vi "sub_check_and_autocreate_channel.vi"(8 "error in (no error)":errorcluster, 9 "daq.io Device Channel Label":string, 10 "daq.io Device Channel Key to write to":string, 11 "daq.io type in in":T1) -> (0 "error out":errorcluster, 1 "channel ID":string, 3 "daq.io type out":T1)   [LabVIEW 2013, in "daqio minimal.lvlib"]
doc: "This VI autocreates a new channel type if required."
uses:
  daqio minimal.lvlib
  _typedefs/daqio-Type.ctl
  <vilib>/httpClient/ClientHandle.ctl
  _typedefs/FGV_commands.ctl
  _typedefs/daqio-Channel-Type.ctl
  <vilib>/httpClient/LabVIEWHTTPClient.lvlib
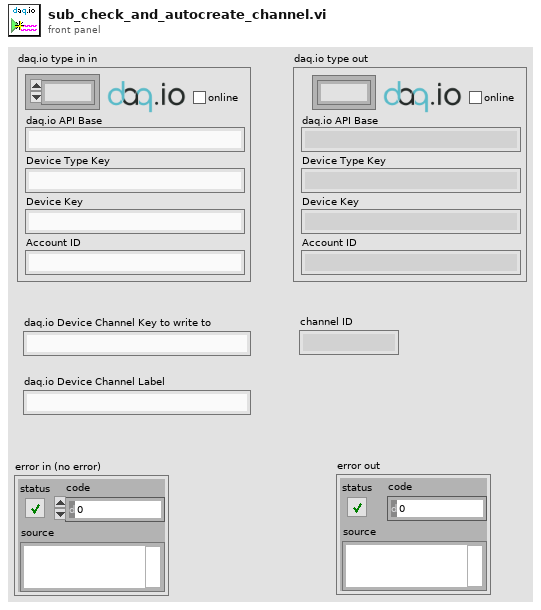
[diagram p1: front panel]
types:
  T1 = typedef "daqio minimal.lvlib/daqio-Type.ctl" = cluster{"daq.io ref":T2, "daq.io API Base":string, "Device Type Key":string, "Device Key":string, "Account ID":string, "online":bool}
  T2 = typedef "LabVIEWHTTPClient.lvlib/ClientHandle.ctl" = refnum<k1>
  T3 = typedef "daqio minimal.lvlib/FGV_commands.ctl" = enum16{"Init / update", "Edit Item", "Find or Add Item", "Remove Item", "Delete All"}
  T4 = typedef "daqio minimal.lvlib/daqio-Channel-Type.ctl" = cluster{"key":string, "label":string, "data_type":string}
  T5 = typedef "daqio minimal.lvlib/daqio-Device-Type-Info-return.ctl" = cluster{"channel_types":T6[], "devices":T7[], "label":string, "event_types":T8[], "key":string, "tag_types":T9[], "id":string, "permissions":cluster{"write":string[], "read":string[]}}
  T6 = typedef "daqio minimal.lvlib/daqio-Channel-Type-POST-return.ctl" = cluster{"device_type_id":string, "id":string, "key":string, "label":string, "data_type":string, "permissions":cluster{"write":string[], "read":string[]}}
  T7 = typedef "daqio minimal.lvlib/daqio-Device.ctl" = cluster{"permissions":cluster{"write":string[], "read":string[]}, "id":string, "label":string, "key":string, "device_type_id":string, "tags":cluster{"key":string, "value":string}[], "files":string[]}
  T8 = typedef "daqio minimal.lvlib/daqio-Event-Type.ctl" = cluster{"device_type_id":string, "permissions":cluster{"read":string[], "write":string[]}, "id":string, "key":string, "label":string}
  T9 = typedef "daqio minimal.lvlib/daqio-Tag-Type-POST-return.ctl" = cluster{"label":string, "id":string, "device_type_id":string, "permissions":cluster{"write":string[], "read":string[]}, "default":string, "key":string}
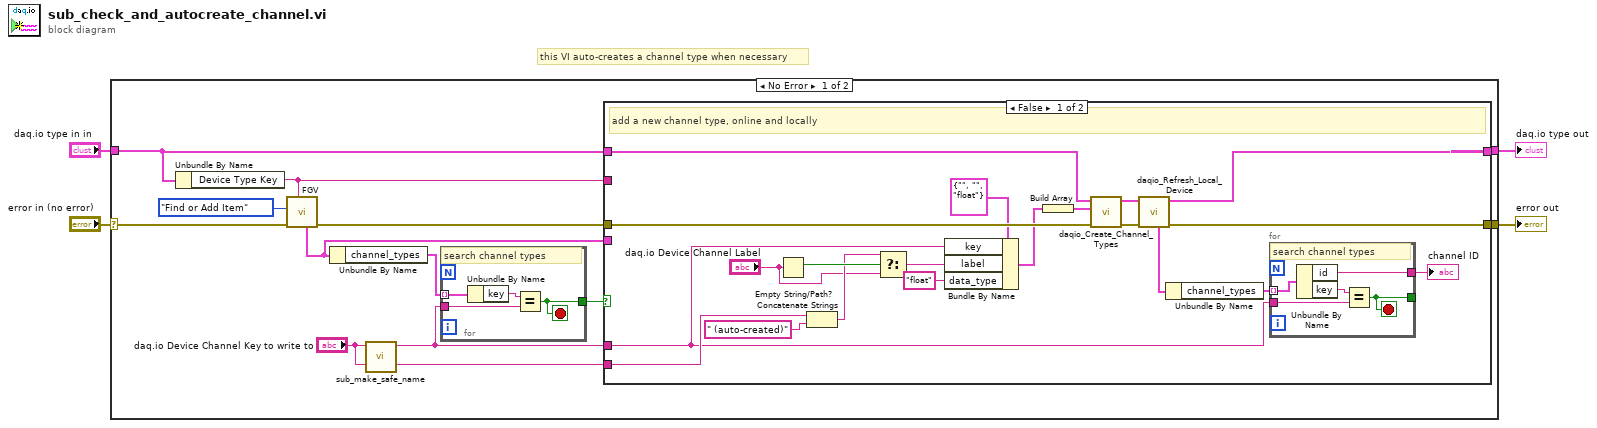
[diagram p0: block diagram]
diagram:
  # "this VI auto-creates a channel type when necessary"
  n1 = case shown="No Error" "error in (no error)" {
    selector: "error in (no error)" -> [w8 w49]
    tunnel: [w10 w49] -> w4
    tunnel: [w9 w48] -> w3
    tunnel: "daq.io type in in" -> [w7 w48]
    frame No Error {
      n2 = Unbundle By Name(w7) -> ("Device Type Key"=w6:string)
      n3 = call "FGV.vi"("Dev Type Key"=w6, "error in (no error)"=w8, "Action"=FGV_commands."Find or Add Item") -> ("error out"=w14:errorcluster, "Dev Type out"=w15:T5)  [unwired: 4 in, 3 out]
      n4 = Unbundle By Name(w15) -> ("channel_types"=w12:T6[])
      n5 = call "sub_make_safe_name.vi"("Input String"="daq.io Device Channel Key to write to") -> ("Safe Output String"=w16:string)  [unwired: 10 in]
      n6 = for {
        tunnel: w12 -> [w47] mode=indexing
        tunnel: w16 -> [w45]
        tunnel: [w44] -> w13
        stop <- w44 stop-if-true
        # "search channel types"
        n7 = Unbundle By Name(w47) -> ("key"=w46:string)
        n8 = Equal?(x=w46, y=w45) -> (x = y?=w44:bool)
      }
      n9 = case shown="False" w13 {
        tunnel: w7 -> [w27 w43]
        tunnel: [w31 w43] -> w9
        tunnel: w16 -> [w18 _]
        tunnel: w14 -> [w33 w42]
        tunnel: [w32 w42] -> w10
        tunnel: w6 -> [_ _]
        tunnel: w15 -> [_ _]
        tunnel: "daq.io Device Channel Key to write to" -> [w26 _]
        frame False {
          # "add a new channel type, online and locally"
          n10 = Empty String/Path?(string/path="daq.io Device Channel Label") -> (empty?=w24:bool)
          n11 = Concatenate Strings(w26, " (auto-created)" ("string")) -> (w23:string)
          n12 = Select(t=w23, s=w24, f="daq.io Device Channel Label") -> (s? t:f=w21:string)
          n13 = Bundle By Name(cluster=T4 {"key"="", "label"="", "data_type"="float"} ("channel type"), "key"=w18, "label"=w21, "data_type"="float") -> (w29:T4)
          n14 = Build Array(w29) -> (w28:T4[])
          n15 = call "daqio_Create_Channel_Types.vi"("error in (no error)"=w33, "Channel Types"=w28, "daq.io type in"=w27) -> ("error out"=w34:errorcluster, "daq.io type out"=w35:T1)  [unwired: 7 in]
          n16 = call "daqio_Refresh_Local_Device.vi"("error in (no error)"=w34, "daq.io type in"=w35) -> ("error out"=w32:errorcluster, "daq.io type out"=w31:T1, "Dev Type out"=w20:T5)  [unwired: 5 in, 2 out]
          n17 = Unbundle By Name(w20) -> ("channel_types"=w19:T6[])
          n18 = for {
            tunnel: w19 -> [w41] mode=indexing
            tunnel: w18 -> [w39]
            tunnel: [w38] -> _
            tunnel: [w37] -> w17
            stop <- w38 stop-if-true
            # "search channel types"
            n19 = Unbundle By Name(w41) -> ("id"=w37:string, "key"=w40:string)
            n20 = Equal?(x=w40, y=w39) -> (x = y?=w38:bool)
          }
          "channel ID" <- w17
        }
        frame True {
          # "don't add anything, it exists"
        }
      }
    }
    frame Error {
    }
  }
  "error out" <- w4
  "daq.io type out" <- w3
